vi "ADC_V6_Global .vi"() -> ()   [LabVIEW 2015]
uses:
  E:/P1_ADC_TEST_2017/LabVIEW_1130/LBNE_DLL/LBNE_DLL/bin/Debug/LBNE_DLL.dll
panel:
  out "DUNE_REF":refnum<k24>
  out "UDP/I2C 2":bool
  out "UDP/I2C":bool
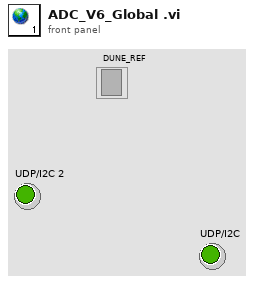
[diagram p1: front panel]
diagram:
